vi "Library Read Text File.vi"(0 "file path":path, 1 "convert eol (F)":bool, 11 "error in (no error)":errorcluster) -> (4 "dup path":path, 8 "read text":string, 15 "error out":errorcluster)   [LabVIEW 2012]
doc: "Reads a text file with optional eol conversion."
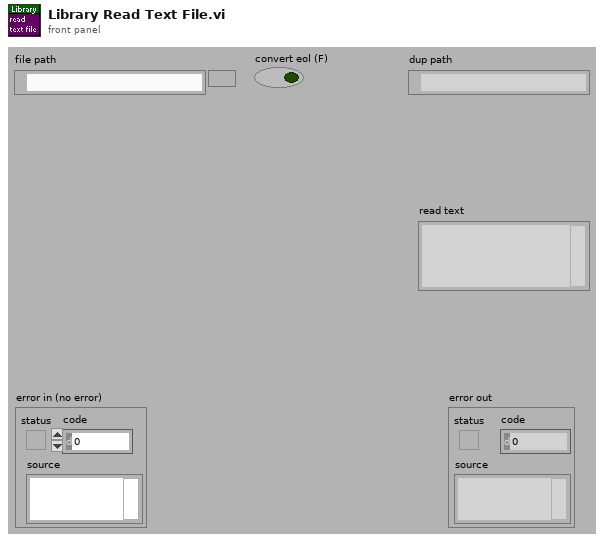
[diagram p1: front panel]
types:
  T1 = enum16{"deny read/write", "deny write-only", "deny none"}
  T2 = enum16{"read/write", "read-only", "write-only", "write-only (truncate)"}
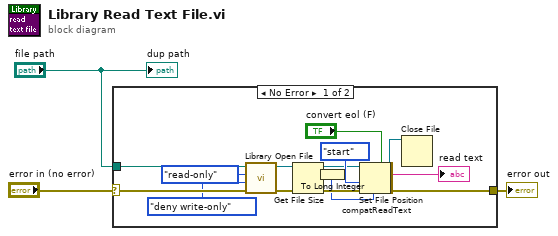
[diagram p0: block diagram]
diagram:
  n1 = case shown="No Error" "error in (no error)" {
    selector: "error in (no error)" -> [w11 w21]
    tunnel: [w12 w21] -> w3
    tunnel: "file path" -> [w8 _]
    frame No Error {
      n2 = call "Library Open File.vi"("error in (no error)"=w11, "deny mode (deny none)"=T1."deny write-only", "open mode (read/write)"=T2."read-only", "file path"=w8) -> ("error out"=w14:errorcluster, "refnum"=w13:refnum<file>)  [unwired: 2 in]
      n3 = Get File Size(file=w13, error in=w14) -> (refnum out=w18:refnum<file>, size (in bytes)=w6:i64, 0:w17:errorcluster)
      n4 = To Long Integer(number=w6) -> (32bit integer=w16:i32)
      n5 = Set File Position(refnum=w18, from (0:start)=enum16{"start", "end", "current"}."start" ("pos mode (0:2)"), error in=w17) -> (refnum out=w5:refnum<file>, error out=w4:errorcluster)  [unwired: 1 in]
      n6 = call <vilib>:"compatReadText.vi"("convert eol (F)"="convert eol (F)", "count"=w16, "error in"=w4, "refnum"=w5) -> ("error out"=w12:errorcluster, "data"=→"read text":string, "dup refnum"=w15:refnum<file>)  [unwired: 5 in]
      n7 = Close File(refnum=w15) -> ()  [unwired: 1 in, 2 out]
    }
    frame Error {
    }
  }
  "error out" <- w3
  "dup path" <- "file path"
